vi "SSH Execute Command.vi"(8 "Error In":errorcluster, 10 "Command":string, 11 "SSH Session":refnum<k1>) -> (0 "Error Out":errorcluster, 2 "Std Out":string, 3 "SSH Session":refnum<k1>)   [LabVIEW 2020, in "LMH-LINX.lvlib"]
uses:
  LMH-LINX.lvlib
  C:/Users/rkalbermatter/Projects/LabVIEW Hobbyist/LINX/LabVIEW/vi.lib/MakerHub/LINX/Resources/Renci.SshNet.dll
  Resources/Renci.SshNet.dll
  SSH Unix Session Op.ctl
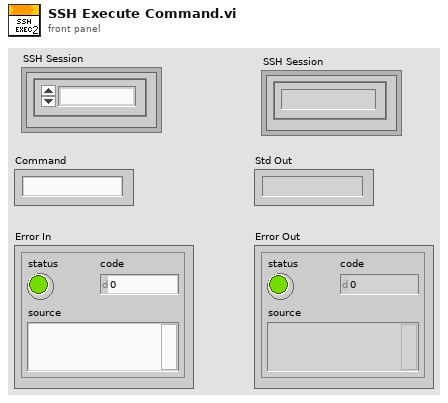
[diagram p1: front panel]
types:
  T1 = typedef "LMH-LINX.lvlib/SSH Unix Session Op.ctl" = enum16{"New", "Get", "Delete"}
  T2 = typedef "LMH-LINX.lvlib/SSH Unix Session Info.ctl" = cluster{"PID":i32, "Read FD":i32, "Write FD":i32, "Error FD":i32}
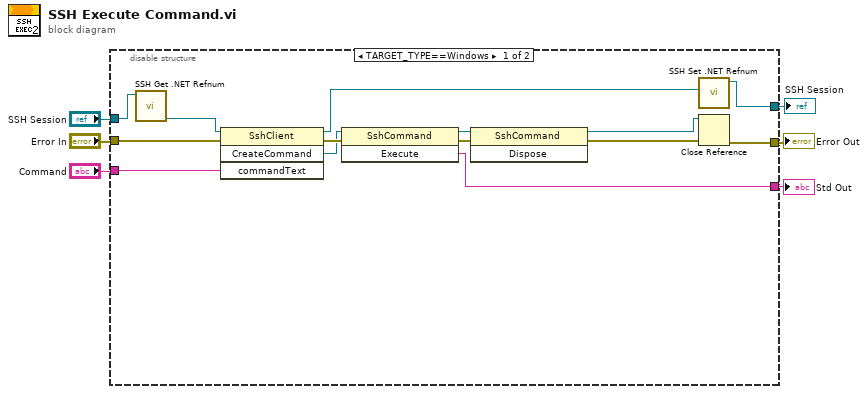
[diagram p0: block diagram]
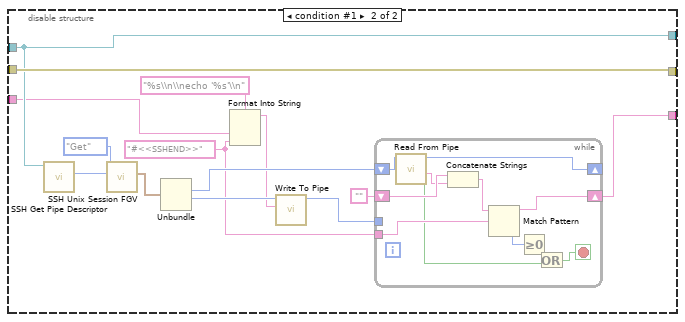
[diagram p2: hidden frame]
diagram:
  n1 = disable-structure shown="TARGET_TYPE==Windows" {
    disable-tunnel: [w17 w21] -> w2
    disable-tunnel: "SSH Session" -> [w9 w33]
    disable-tunnel: "Error In" -> [w16 w34]
    disable-tunnel: "Command" -> [w15 w27]
    disable-tunnel: [w7 w33] -> w1
    disable-tunnel: [w12 w34] -> w3
    frame condition #0 (active) {
      n2 = call "SSH Get .NET Refnum.vi"("SSH Session"=w9) -> ("SSH .NET Refnum"=w10:refnum<k24>)  [unwired: 8 in, 2 out]
      n3 = invoke class="SshClient" method="CreateCommand"(reference=w10, error in=w16, "commandText"=w15) -> (reference out=w8:refnum<k24>, error out=w20:errorcluster, "CreateCommand"=w14:refnum<k24>)  [unwired: 1 in, 1 out]
      n4 = invoke class="SshCommand" method="Execute"(reference=w14, error in=w20) -> (reference out=w19:refnum<k24>, error out=w18:errorcluster, "Execute"=w17:string)  [unwired: 1 in]
      n5 = invoke class="SshCommand" method="Dispose"(reference=w19, error in=w18) -> (reference out=w11:refnum<k24>, error out=w13:errorcluster)  [unwired: 1 in, 1 out]
      n6 = call "SSH Set .NET Refnum.vi"("SSH .NET Refnum"=w8) -> ("SSH Session"=w7:refnum<k1>)  [unwired: 9 in, 1 out]
      n7 = Close Reference(reference=w11, error in (no error)=w13) -> (error out=w12:errorcluster)
    }
    frame condition #1 {
      w23 = "#<<SSHEND>>"
      n8 = call "SSH Get Pipe Descriptor.vi"("SSH Session"=w33) -> ("SSH Pipe Descriptor"=w31:i32)  [unwired: 8 in, 2 out]
      n9 = call "SSH Unix Session FGV.vi"("Session In"=w31, "Operation"=SSH_Unix_Session_Op."Get") -> ("info in"=w30:T2)  [unwired: 8 in, 1 out]
      n10 = Unbundle(w30) -> ("Read FD"=w28:i32, "Write FD"=w29:i32)  [unwired: 2 out]
      n11 = Format Into String(format string="%s\\n\\necho '%s'\\n", w27, w23) -> (resulting string=w26:string)  [unwired: 2 in, 1 out]
      n12 = call <vilib>:"Write To Pipe.vi"("data"=w26, "file descriptor"=w29) -> ("file descriptor"=w24:i32)  [unwired: 3 in, 2 out]
      n13 = while {
        shift-right: [w44] -> _
        shift-left: w28 -> [w45]
        tunnel: w24 -> [_]
        tunnel: w23 -> [w43]
        shift-right: [w39] -> w21
        shift-left: "" -> [w42]
        stop <- w37 stop-if-true
        n14 = call <vilib>:"Read From Pipe.vi"("file descriptor"=w45) -> ("eof?"=w35:bool, "file descriptor"=w44:i32, "data"=w41:string)  [unwired: 3 in, 2 out]
        n15 = Concatenate Strings(w42, w41) -> (w40:string)
        n16 = Match Pattern(string=w40, regular expression=w43) -> (before substring=w39:string, offset past match=w38:i32)  [unwired: 1 in, 2 out]
        n17 = Greater Or Equal To 0?(x=w38) -> (x >= 0?=w36:bool)
        n18 = Or(x=w36, y=w35) -> (x .or. y?=w37:bool)
      }
    }
  }
  "Error Out" <- w3
  "Std Out" <- w2
  "SSH Session" <- w1
